vi "NML VISA Bus Scan.vi"() -> (0 "Instrument List":T1[](array[typedef]) {"Status" format="%.0x"})   [LabVIEW 2019]
doc: "Scans all primary addresses on the GPIB bus and reports status of devices found there.\nScott Hannahs, F. Bitter National Magnet Lab, April 1993"
uses:
  Sub Controls/Instrument IDN.ctl
  Sub Controls/Instrument Ref.ctl
  SubVIs/SetupGlobals.vi
panel:
  out "Extra Info":i32[](array[numeric])
  out "error out":errorcluster
  # "VISA Address"
  # "Status"
  # "Manufacturer"
  # "Model"
  # "Serial Number"
  # "Firmware"
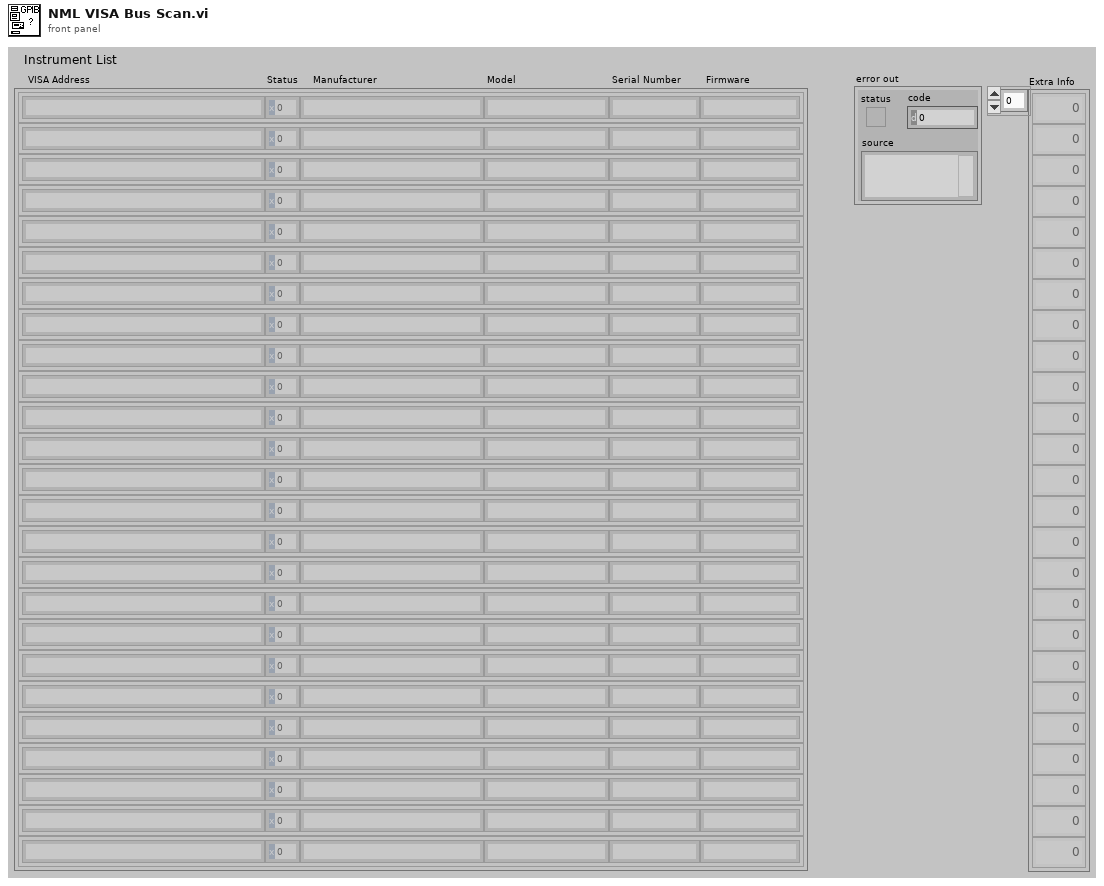
[diagram p1: front panel]
types:
  T1 = typedef "Instrument IDN.ctl" = cluster{"VISA Address":string, "Status":u16, "Manufacturer":string, "Model":string, "Info":string, "Info 2":string, "Misc Data":variant}
  T2 = typedef "Instrument Ref.ctl" = refnum<vi>
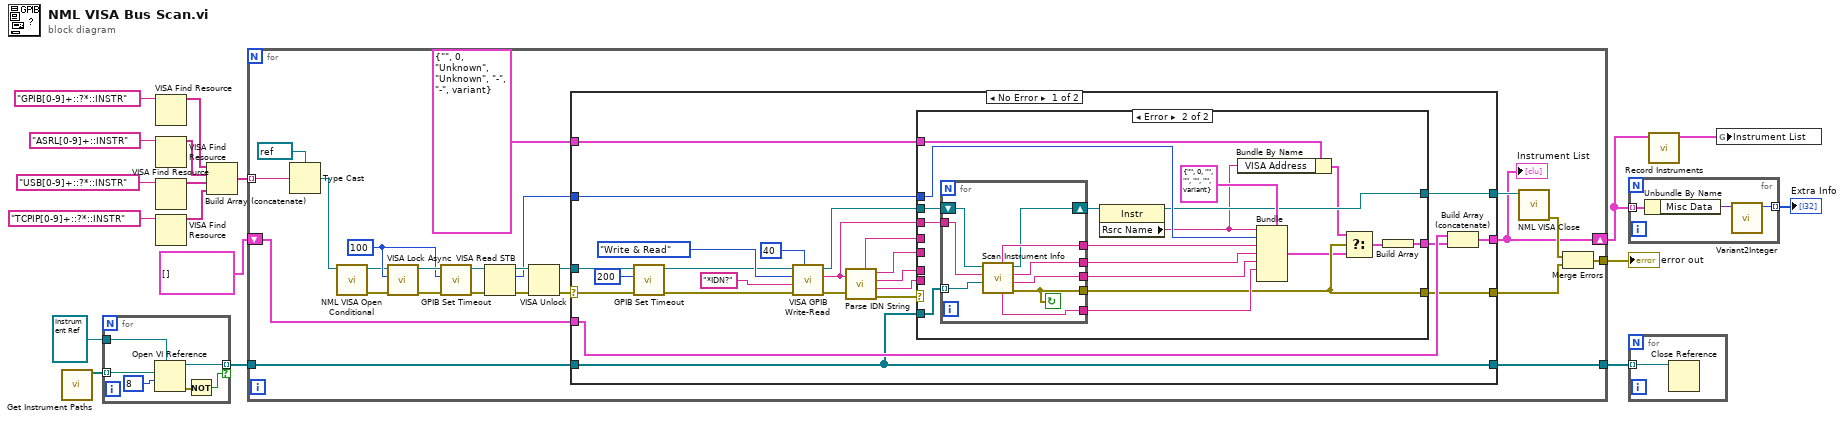
[diagram p0: block diagram]
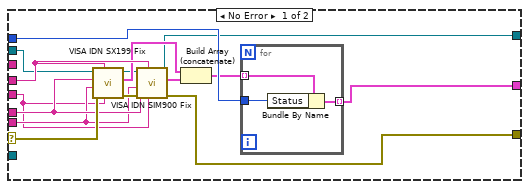
[diagram p2: hidden frame]
diagram:
  n1 = call "Get Instrument Paths.vi"() -> ("paths"=w12:path[])  [unwired: 1 in]
  n2 = for {
    tunnel: w12 -> [w24] mode=indexing
    tunnel: [w22] -> w15 mode=indexing if=w19
    tunnel: T2 refnum ("Private.VI Refnum") -> [w23]
    n3 = Open VI Reference(type specifier VI Refnum (for type only)=w23, vi path=w24, options=8) -> (vi reference=w22:T2, error out=w20:errorcluster)  [unwired: 3 in]
    n4 = Not(x=w20) -> (.not. x?=w19:bool)
  }
  n5 = VISA Find Resource(11:"GPIB[0-9]+::?*::INSTR" ("expression (\"?*\")")) -> (3:w4:string[])  [unwired: 2 in, 2 out]
  n6 = VISA Find Resource(11:"ASRL[0-9]+::INSTR" ("expression (\"?*\")")) -> (3:w5:string[])  [unwired: 2 in, 2 out]
  n7 = VISA Find Resource(11:"USB[0-9]+::?*::INSTR" ("expression (\"?*\")")) -> (3:w6:string[])  [unwired: 2 in, 2 out]
  n8 = VISA Find Resource(11:"TCPIP[0-9]+::?*::INSTR" ("expression (\"?*\")")) -> (3:w16:string[])  [unwired: 2 in, 2 out]
  n9 = Build Array (concatenate)(w4, w5, w6, w16) -> (w7:string[])
  n10 = for {
    tunnel: w7 -> [w40] mode=indexing
    tunnel: [w31] -> w18
    shift-right: [w42] -> w1
    shift-left: T1[] [] ("Instrument List") -> [w44]
    tunnel: w15 -> [w34]
    tunnel: [w33] -> w13
    w35 = u32 100 ("General Settings:Timeout Value")
    n11 = Type Cast(type=refnum<visa-resource-name> refnum ("VISA resource name out"), x=w40) -> (*(type *) &x=w26:refnum<visa-resource-name>)
    n12 = call "NML VISA Open Conditional.vi"("VISA resource name"=w26) -> ("error out"=w28:errorcluster, "dup VISA Session"=w27:refnum<visa-resource-name>)  [unwired: 8 in, 1 out]
    n13 = call <vilib>:"VISA Lock Async.vi"("error in (no error)"=w28, "timeout (0)"=w35, "VISA resource name"=w27) -> ("error out"=w36:errorcluster, "VISA resource name out"=w37:refnum<visa-resource-name>)  [unwired: 6 in, 1 out]
    n14 = call "GPIB Set Timeout.vi"("Error In"=w36, "Timeout"=w35, "VISA resource name"=w37) -> ("Error Out"=w41:errorcluster, "dup VISA resource name"=w47:refnum<visa-resource-name>)  [unwired: 2 in, 1 out]
    n15 = VISA Read STB(8:w41, 11:w47) -> (0:w29:errorcluster, 2:w43:u16, 3:w46:refnum<visa-resource-name>)
    n16 = VISA Unlock(8:w29, 11:w46) -> (0:w38:errorcluster, 3:w39:refnum<visa-resource-name>)
    n17 = case shown="No Error" w38 {
      selector: w38 -> [w57 w120]
      tunnel: [w68 w120] -> w30
      tunnel: w39 -> [w58 w121]
      tunnel: [w52 w121] -> w45
      tunnel: w44 -> [w71 w119]
      tunnel: [w72 w119] -> w42
      tunnel: w43 -> [w51 _]
      tunnel: w34 -> [w59 w118]
      tunnel: [w59 w118] -> w33
      tunnel: T1 {"VISA Address"="", "Status"=0, "Manufacturer"="Unknown", "Model"="Unknown", "Info"="-", "Info 2"="-", "Misc Data"=variant} ("t") -> [w49 _]
      frame No Error {
        n18 = call "GPIB Set Timeout.vi"("Error In"=w57, "Timeout"=u32 200 ("General Settings:Timeout Value"), "VISA resource name"=w58) -> ("Error Out"=w56:errorcluster, "dup VISA resource name"=w55:refnum<visa-resource-name>)  [unwired: 2 in, 1 out]
        n19 = call "VISA GPIB Write-Read.vi"("Wait (ms)"=u32 40 ("wait (mS)"), "error in (no error)"=w56, "Command"="*IDN?" ("write buffer (\"\")"), "Action"=enum16{"Write", "Read", "Write & Read"}."Write & Read", "VISA resource name"=w55) -> ("error out"=w70:errorcluster, "String Returned"=w62:string, "dup VISA Session"=w63:refnum<visa-resource-name>)  [unwired: 3 in, 1 out]
        n20 = call "Parse IDN String.vi"("error in (no error)"=w70, "IDN String"=w62) -> ("error out"=w69:errorcluster, "Info"=w67:string, "Model"=w66:string, "Manufacturer"=w65:string, "Revision"=w64:string)
        n21 = case shown="Error" w69 {
          selector: w69 -> [w86 _]
          tunnel: [w83 w96] -> w68
          tunnel: w67 -> [w79 _]
          tunnel: w66 -> [w80 _]
          tunnel: w65 -> [w76 _]
          tunnel: w64 -> [w81 _]
          tunnel: [w73 w97] -> w52
          tunnel: w59 -> [_ w108]
          tunnel: w63 -> [w78 w107]
          tunnel: w62 -> [_ w106]
          tunnel: w51 -> [w85 w103]
          tunnel: [w84 w104] -> w50
          tunnel: w49 -> [_ w93]
          frame No Error {
            n22 = call "VISA IDN SX199 Fix.vi"("Manufacturer in"=w76, "Revision in"=w81, "error in (no error)"=w86, "Info in"=w79, "Model in"=w80, "VISA Resource Name"=w78) -> ("error out"=w87:errorcluster, "Devices"=w77:T1[], "dup VISA Session"=w75:refnum<visa-resource-name>)  [unwired: 2 in, 1 out]
            n23 = call "VISA IDN SIM900 Fix.vi"("Manufacturer in"=w76, "Revision in"=w81, "error in (no error)"=w87, "Info in"=w79, "Model in"=w80, "VISA Resource Name"=w75) -> ("error out"=w83:errorcluster, "Devices"=w74:T1[], "dup VISA Session"=w73:refnum<visa-resource-name>)  [unwired: 3 in]
            n24 = Build Array (concatenate)(w77, w74) -> (w82:T1[])
            n25 = for {
              tunnel: w82 -> [w90] mode=indexing
              tunnel: w85 -> [w89]
              tunnel: [w88] -> w84 mode=indexing
              n26 = Bundle By Name(cluster=w90, "Status"=w89) -> (w88:T1)
            }
          }
          frame Error {
            n27 = for {
              tunnel: w108 -> [w116] mode=indexing
              tunnel: w106 -> [w117]
              tunnel: [w115] -> w102
              tunnel: [w110] -> w99
              tunnel: [w114] -> w100
              tunnel: [w113] -> w101
              tunnel: [w111] -> w96
              shift-right: [w109] -> w98
              shift-left: w107 -> [w112]
              stop <- w111 continue-if-true
              n28 = call "Scan Instrument Info.vi"("VISA resource name"=w112, "ID String in"=w117, "Private.VI Refnum"=w116) -> ("Manufacturer"=w110:string, "Revision"=w115:string, "VISA resource name Out"=w109:refnum<visa-resource-name>, "Model"=w114:string, "Info"=w113:string, "error out"=w111:errorcluster)  [unwired: 1 in]
            }
            n29 = property class="Instr"(reference=w98) -> (reference out=w97:refnum<visa-resource-name>, "Rsrc Name"=w91:string)  [unwired: 1 in, 1 out]
            n30 = Bundle By Name(cluster=w93, "VISA Address"=w91) -> (w92:T1)
            n31 = Bundle(cluster=T1 {"VISA Address"="", "Status"=0, "Manufacturer"="", "Model"="", "Info"="", "Info 2"="", "Misc Data"=variant} ("Instrument List"), "VISA Address"=w91, "Status"=w103, "Manufacturer"=w99, "Model"=w100, "Info"=w101, "Info 2"=w102) -> (w95:T1)  [unwired: 1 in]
            n32 = Select(t=w92, s=w96, f=w95) -> (s? t:f=w94:T1)
            n33 = Build Array(w94) -> (w104:T1[])
          }
        }
        n34 = Build Array (concatenate)(w71, w50) -> (w72:T1[])
      }
      frame Error {
      }
    }
    "Instrument List" <- w42
    n35 = call "NML VISA Close.vi"("VISA resource name"=w45) -> ("Error Out"=w48:errorcluster)  [unwired: 10 in]
    n36 = Merge Errors(w48, w30) -> (w31:errorcluster)
  }
  "error out" <- w18
  n37 = for {
    tunnel: w1 -> [w124] mode=indexing
    tunnel: [w123] -> w3 mode=indexing
    n38 = Unbundle By Name(w124) -> ("Misc Data"=w122:variant)
    n39 = call "Variant2Integer.vi"("Variant"=w122) -> ("data"=w123:i32)  [unwired: 9 in, 1 out]
  }
  "Extra Info" <- w3
  n40 = for {
    tunnel: w13 -> [w125] mode=indexing
    n41 = Close Reference(reference=w125) -> ()  [unwired: 1 in, 1 out]
  }
  n42 = call "Record Instruments.vi"("Instrument List in"=w1) -> ("Instrument List out"=w2:T1[])  [unwired: 9 in, 1 out]
  n43 = global write "SetupGlobals.vi" "Instrument List"(w2) -> ()
